vi "Read Write Header.vi"(0 "Header Table 1 IN":string[][](array[string]), 1 "Header Table 2 IN":string[][](array[string]), 2 "Sys Cal Table IN":string[][](array[string]), 3 "Cal Standards Table IN":string[][](array[string]), 4 "Header Comments IN":string[][](array[string]), 6 "Cal Template Path":path, 8 "Write (F)":bool) -> (14 "Header Table 1":string[][](array[string]), 15 "Header Table 2":string[][](array[string]), 16 "Sys Cal Table":string[][](array[string]), 17 "Cal Standards Table":string[][](array[string]), 18 "Header Comments":string[][](array[string]))   [LabVIEW 2019]
uses:
  Type Defs/Excel Driver Operator Type Def.ctl
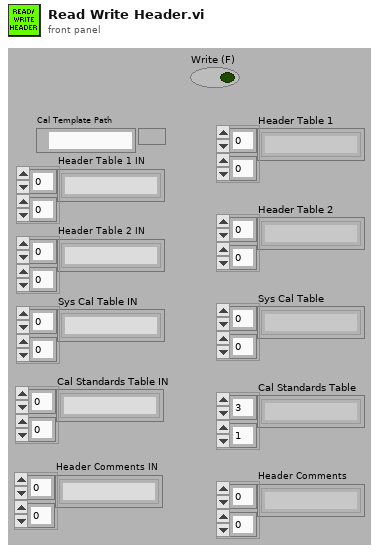
[diagram p1: front panel]
types:
  T1 = typedef "Excel Driver Operator Type Def.ctl" = enum16{"Open", "Close", "Search for String", "GetUsedRange", "Read Range", "Read Cell", "Set Range", "Set Cell"}
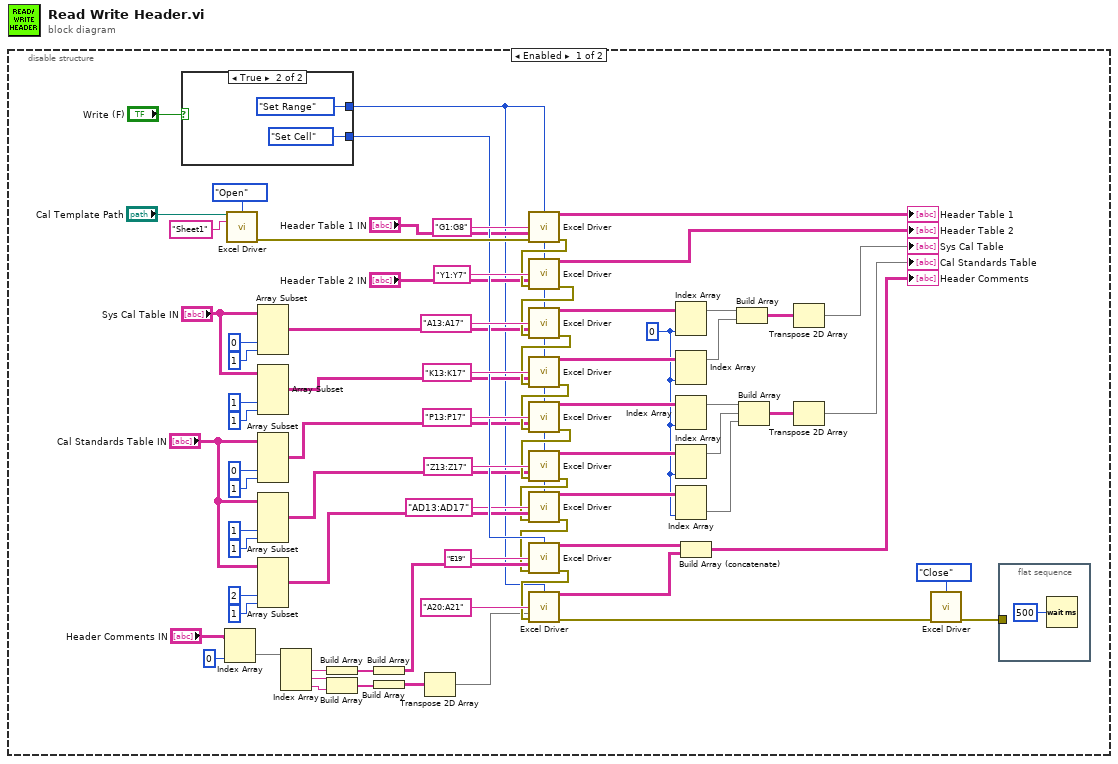
[diagram p0: block diagram]
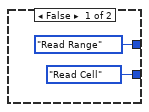
[diagram p2: hidden frame]
diagram:
  n1 = disable-structure shown="Enabled" {
    frame Enabled {
      w4 = 0 ("disabled index (col)")
      n2 = case shown="True" "Write (F)" {
        tunnel: [Excel_Driver_Operator_Type_Def."Read Range" ("Operator") Excel_Driver_Operator_Type_Def."Set Range" ("Operator")] -> w1
        tunnel: [Excel_Driver_Operator_Type_Def."Read Cell" ("Operator") Excel_Driver_Operator_Type_Def."Set Cell" ("Operator")] -> w39
        frame False {
        }
        frame True {
        }
      }
      n3 = Index Array(array="Header Comments IN", index (col)=0 ("disabled index (col)")) -> (element=w24:string[])  [unwired: 1 in]
      n4 = call "Excel Driver.vi"("Filename of Workbook"="Cal Template Path", "Operator"=Excel_Driver_Operator_Type_Def."Open", "WorkSheet Name"="Sheet1") -> ("error out"=w51:errorcluster)  [unwired: 10 in, 2 out]
      n5 = Array Subset(array="Sys Cal Table IN", index (col)=0 ("index"), length (col)=1 ("length")) -> (w34:string[][])  [unwired: 2 in]
      n6 = Array Subset(array="Sys Cal Table IN", index (col)=1 ("index"), length (col)=1 ("length")) -> (w15:string[][])  [unwired: 2 in]
      n7 = Array Subset(array="Cal Standards Table IN", index (col)=0 ("index"), length (col)=1 ("length")) -> (w14:string[][])  [unwired: 2 in]
      n8 = Array Subset(array="Cal Standards Table IN", index (col)=1 ("index"), length (col)=1 ("length")) -> (w13:string[][])  [unwired: 2 in]
      n9 = Array Subset(array="Cal Standards Table IN", index (col)=2 ("index"), length (col)=1 ("length")) -> (w6:string[][])  [unwired: 2 in]
      n10 = Index Array(array=w24) -> (element #1=w23:string, element #2=w20:string, element #3=w19:string)  [unwired: 3 in]
      n11 = Build Array(w23) -> (w22:string[])
      n12 = Build Array(w20, w19) -> (w18:string[])
      n13 = Build Array(w22) -> (w21:string[][])
      n14 = Build Array(w18) -> (w17:string[][])
      n15 = Transpose 2D Array(2D array=w17) -> (transposed array=w16:string[][])
      n16 = call "Excel Driver.vi"("Operator"=w1, "Range String\n(Or Search String)"="G1:G8" ("Range String\n(Or Search String)"), "Cell Values INPUT"="Header Table 1 IN", "error in (no error)"=w51) -> ("Cell Values OUT"=→"Header Table 1":string[][], "error out"=w41:errorcluster)  [unwired: 9 in, 1 out]
      n17 = call "Excel Driver.vi"("Operator"=w1, "Range String\n(Or Search String)"="Y1:Y7" ("Range String\n(Or Search String)"), "Cell Values INPUT"="Header Table 2 IN", "error in (no error)"=w41) -> ("Cell Values OUT"=→"Header Table 2":string[][], "error out"=w42:errorcluster)  [unwired: 9 in, 1 out]
      n18 = call "Excel Driver.vi"("Operator"=w1, "Range String\n(Or Search String)"="A13:A17" ("Range String\n(Or Search String)"), "Cell Values INPUT"=w34, "error in (no error)"=w42) -> ("Cell Values OUT"=w57:string[][], "error out"=w43:errorcluster)  [unwired: 9 in, 1 out]
      n19 = call "Excel Driver.vi"("Operator"=w1, "Range String\n(Or Search String)"="K13:K17" ("Range String\n(Or Search String)"), "Cell Values INPUT"=w15, "error in (no error)"=w43) -> ("Cell Values OUT"=w58:string[][], "error out"=w45:errorcluster)  [unwired: 9 in, 1 out]
      n20 = call "Excel Driver.vi"("Operator"=w1, "Range String\n(Or Search String)"="P13:P17" ("Range String\n(Or Search String)"), "Cell Values INPUT"=w14, "error in (no error)"=w45) -> ("Cell Values OUT"=w60:string[][], "error out"=w44:errorcluster)  [unwired: 9 in, 1 out]
      n21 = call "Excel Driver.vi"("Operator"=w1, "Range String\n(Or Search String)"="Z13:Z17" ("Range String\n(Or Search String)"), "Cell Values INPUT"=w13, "error in (no error)"=w44) -> ("Cell Values OUT"=w59:string[][], "error out"=w2:errorcluster)  [unwired: 9 in, 1 out]
      n22 = call "Excel Driver.vi"("Operator"=w1, "Range String\n(Or Search String)"="AD13:AD17" ("Range String\n(Or Search String)"), "Cell Values INPUT"=w6, "error in (no error)"=w2) -> ("Cell Values OUT"=w5:string[][], "error out"=w7:errorcluster)  [unwired: 9 in, 1 out]
      n23 = call "Excel Driver.vi"("Operator"=w39, "Range String\n(Or Search String)"="E19" ("Range String\n(Or Search String)"), "Cell Values INPUT"=w21, "error in (no error)"=w7) -> ("Cell Values OUT"=w65:string[][], "error out"=w46:errorcluster)  [unwired: 9 in, 1 out]
      n24 = call "Excel Driver.vi"("Operator"=w1, "Range String\n(Or Search String)"="A20:A21" ("Range String\n(Or Search String)"), "Cell Values INPUT"=w16, "error in (no error)"=w46) -> ("Cell Values OUT"=w66:string[][], "error out"=w76:errorcluster)  [unwired: 9 in, 1 out]
      n25 = Index Array(array=w57, index (col)=w4) -> (element=w70:string[])  [unwired: 1 in]
      n26 = Index Array(array=w58, index (col)=w4) -> (element=w71:string[])  [unwired: 1 in]
      n27 = Index Array(array=w60, index (col)=w4) -> (element=w72:string[])  [unwired: 1 in]
      n28 = Index Array(array=w59, index (col)=w4) -> (element=w73:string[])  [unwired: 1 in]
      n29 = Index Array(array=w5, index (col)=w4) -> (element=w3:string[])  [unwired: 1 in]
      n30 = Build Array (concatenate)(w65, w66) -> (→"Header Comments":string[][])
      n31 = Build Array(w70, w71) -> (w68:string[][])
      n32 = Build Array(w72, w73, w3) -> (w69:string[][])
      n33 = Transpose 2D Array(2D array=w68) -> (transposed array=→"Sys Cal Table":string[][])
      n34 = Transpose 2D Array(2D array=w69) -> (transposed array=→"Cal Standards Table":string[][])
      n35 = call "Excel Driver.vi"("Operator"=Excel_Driver_Operator_Type_Def."Close", "error in (no error)"=w76) -> ("error out"=w12:errorcluster)  [unwired: 11 in, 2 out]
      n36 = flat-sequence {
        tunnel: w12 -> [_]
        frame #0 {
          n37 = Wait (ms)(milliseconds to wait=u32 500) -> ()  [unwired: 1 out]
        }
      }
    }
    frame Disabled {
    }
  }
